vi "instance count allowed.vi"(8 "error in":errorcluster, 11 "EthernetIP configuration in":refnum<class "EIP Tags Configuration.lvclass">) -> (0 "error out":errorcluster, 2 "instances allowed":i32, 3 "EthernetIP configuration out":refnum<class "EIP Tags Configuration.lvclass">)   [LabVIEW 2013, in "EIP Tags Configuration.lvclass"]
uses:
  EIP Tags Configuration.lvclass
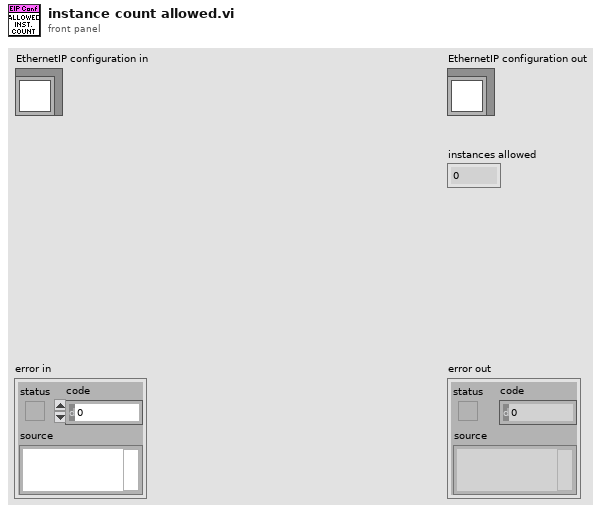
[diagram p1: front panel]
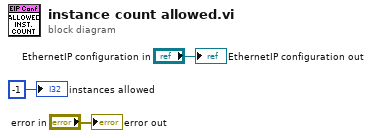
[diagram p0: block diagram]
diagram:
  "error out" <- "error in"
  "EthernetIP configuration out" <- "EthernetIP configuration in"
  "instances allowed" <- -1 ("instances allowed")
